vi "Send Response.vi"(11 "Processing In":refnum<class "Processing.lvclass">) -> (0 "error out":errorcluster, 3 "HTTP Server.lvlib:Processing":refnum<class "Processing.lvclass">)   [LabVIEW 2020, in "HTTP Server.lvlib" / "Server.lvclass"]
uses:
  Server.lvclass
  Processing/Processing.lvclass
  Processing/Processing.lvclass/Processing.ctl
  Server.lvclass/Server.ctl
  lv-http-util/HTTP Utils/Response/Response.lvclass
  RequestTraceLog/RequestTraceLog.lvclass
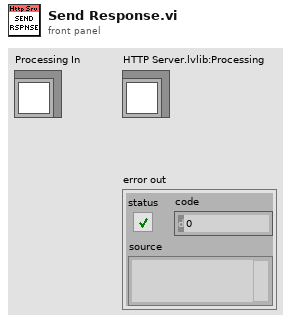
[diagram p1: front panel]
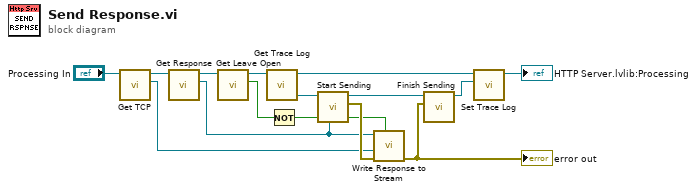
[diagram p0: block diagram]
diagram:
  n1 = call "Get TCP.vi"("Processing in"="Processing In") -> ("TCP"=w1:refnum<k5>, "Processing out"=w7:refnum<class "Processing.lvclass">)  [unwired: 9 in]
  n2 = call "Get Response.vi"("Processing in"=w7) -> ("Response"=w8:refnum<class "Response.lvclass">, "Processing out"=w6:refnum<class "Processing.lvclass">)  [unwired: 9 in]
  n3 = call "Get Leave Open.vi"("Processing in"=w6) -> ("Leave Open"=w3:bool, "Processing out"=w5:refnum<class "Processing.lvclass">)  [unwired: 9 in]
  n4 = call "Get Trace Log.vi"("Processing in"=w5) -> ("Trace Log"=w9:refnum<class "RequestTraceLog.lvclass">, "Processing out"=w4:refnum<class "Processing.lvclass">)  [unwired: 9 in]
  n5 = Not(x=w3) -> (.not. x?=w2:bool)
  n6 = call "Start Sending.vi"("Response"=w8, "RequestTraceLog in"=w9) -> ("error out"=w15:errorcluster, "RequestTraceLog out"=w13:refnum<class "RequestTraceLog.lvclass">)  [unwired: 8 in]
  n7 = call-dynamic "Write Response to Stream.vi"("Close? (T)"=w2, "error in (no error)"=w15, "Stream in"=w1, "Response in"=w8) -> ("error out"=w14:errorcluster)  [unwired: 6 in, 1 out]
  "error out" <- w14
  n8 = call "Finish Sending.vi"("error in (no error)"=w14, "RequestTraceLog in"=w13) -> ("RequestTraceLog out"=w12:refnum<class "RequestTraceLog.lvclass">)  [unwired: 8 in, 1 out]
  n9 = call "Set Trace Log.vi"("Trace Log"=w12, "Processing in"=w4) -> ("Processing out"=→"HTTP Server.lvlib:Processing":refnum<class "Processing.lvclass">)  [unwired: 9 in]
